vi "controleMF.vi"() -> ()   [LabVIEW 2019]
uses:
  <vilib>/Utility/error.llb/DialogType.ctl
  <vilib>/DAQmx/write.llb/DAQmx Write (Counter Frequency 1Chan 1Samp).vi
  <vilib>/DAQmx/create/channels.llb/DAQmx Create Channel (CO-Pulse Generation-Frequency).vi
  <vilib>/DAQmx/configure/timing.llb/DAQmx Timing (Implicit).vi
  <vilib>/DAQmx/miscellaneous.llb/DAQmx Fill In Error Info.vi
  <vilib>/addons/control/pid/pid.llb/PID (DBL).vi
  <vilib>/Utility/file.llb/Write Delimited Spreadsheet (string).vi
  <instrlib>/Agilent 34970/Agilent 34970.lvlib
  <resource>/objmgr/daqmx.rc
  <vilib>/addons/control/pid/NI_PID_pid.lvlib
panel:
  in  "SP:":dbl(slide)=25.0 min=0.0 max=0.0 scale=25.0..50.0
  out "MV":dbl(graph)
  in  "Ts":dbl=1.0
  out "PV":dbl
  out "Process variable and Setpoint":cluster{"initial PV":dbl, "SP:":dbl}(graph)
  in  "PID gains":T1={"proportional gain (Kc)"=39.6, "integral time (Ti, min)"=14.617, "derivative time (Td, min)"=0.0} {"derivative time (Td, min)" format="%.3f"; "integral time (Ti, min)" format="%.3f"; "proportional gain (Kc)" format="%.6f"}
  in  "Frequency":dbl=1.0 format="%.6f"
  out "Duty Cycle":sgl=0.1 min=0.1 max=99.9 format="%#_6f"
  in  "Forno_on":bool=TRUE
  out "Iteration":i32
  out "Chart PV, SP":cluster{dbl, dbl}(graph)
  in  "STOP":bool
  out "Temperature CH4 [degC]":dbl
  out "Temperature CH9 [degC]":dbl
  out "Time":dbl=300.0 format="%<%H:%M:%S>t"
  in  "Identifier":string="ensaioForno"
  # "Geral"
  # "Respostas do Sistema em Malha Fechada"
  # "Controles"
  # "Medidas"
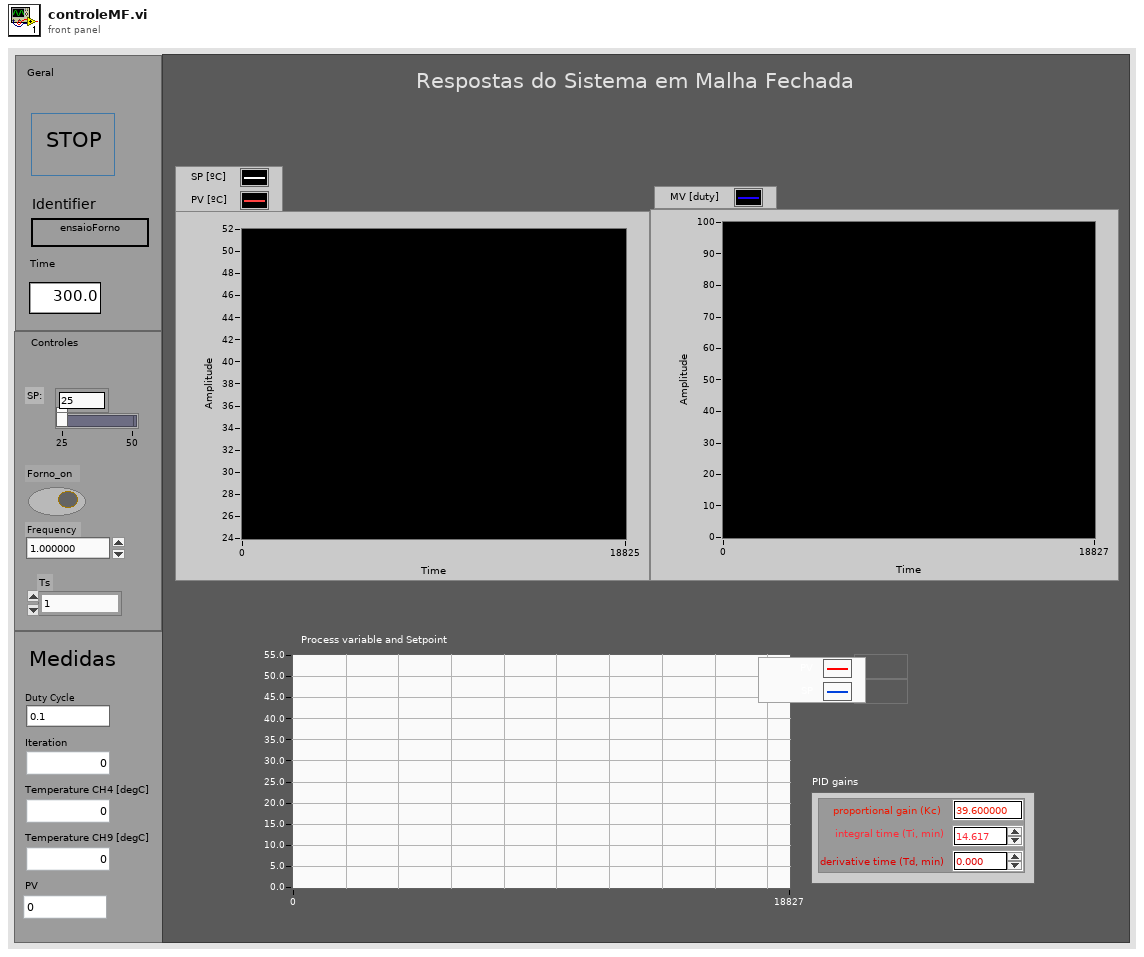
[diagram p1: front panel]
types:
  T1 = cluster{"proportional gain (Kc)":dbl, "integral time (Ti, min)":dbl, "derivative time (Td, min)":dbl}
  T2 = enum16{"Thermocouple", "Thermistor", "RTD", "4-Wire RTD", "Default (Last)"}
  T3 = typedef "DialogType.ctl" = u16
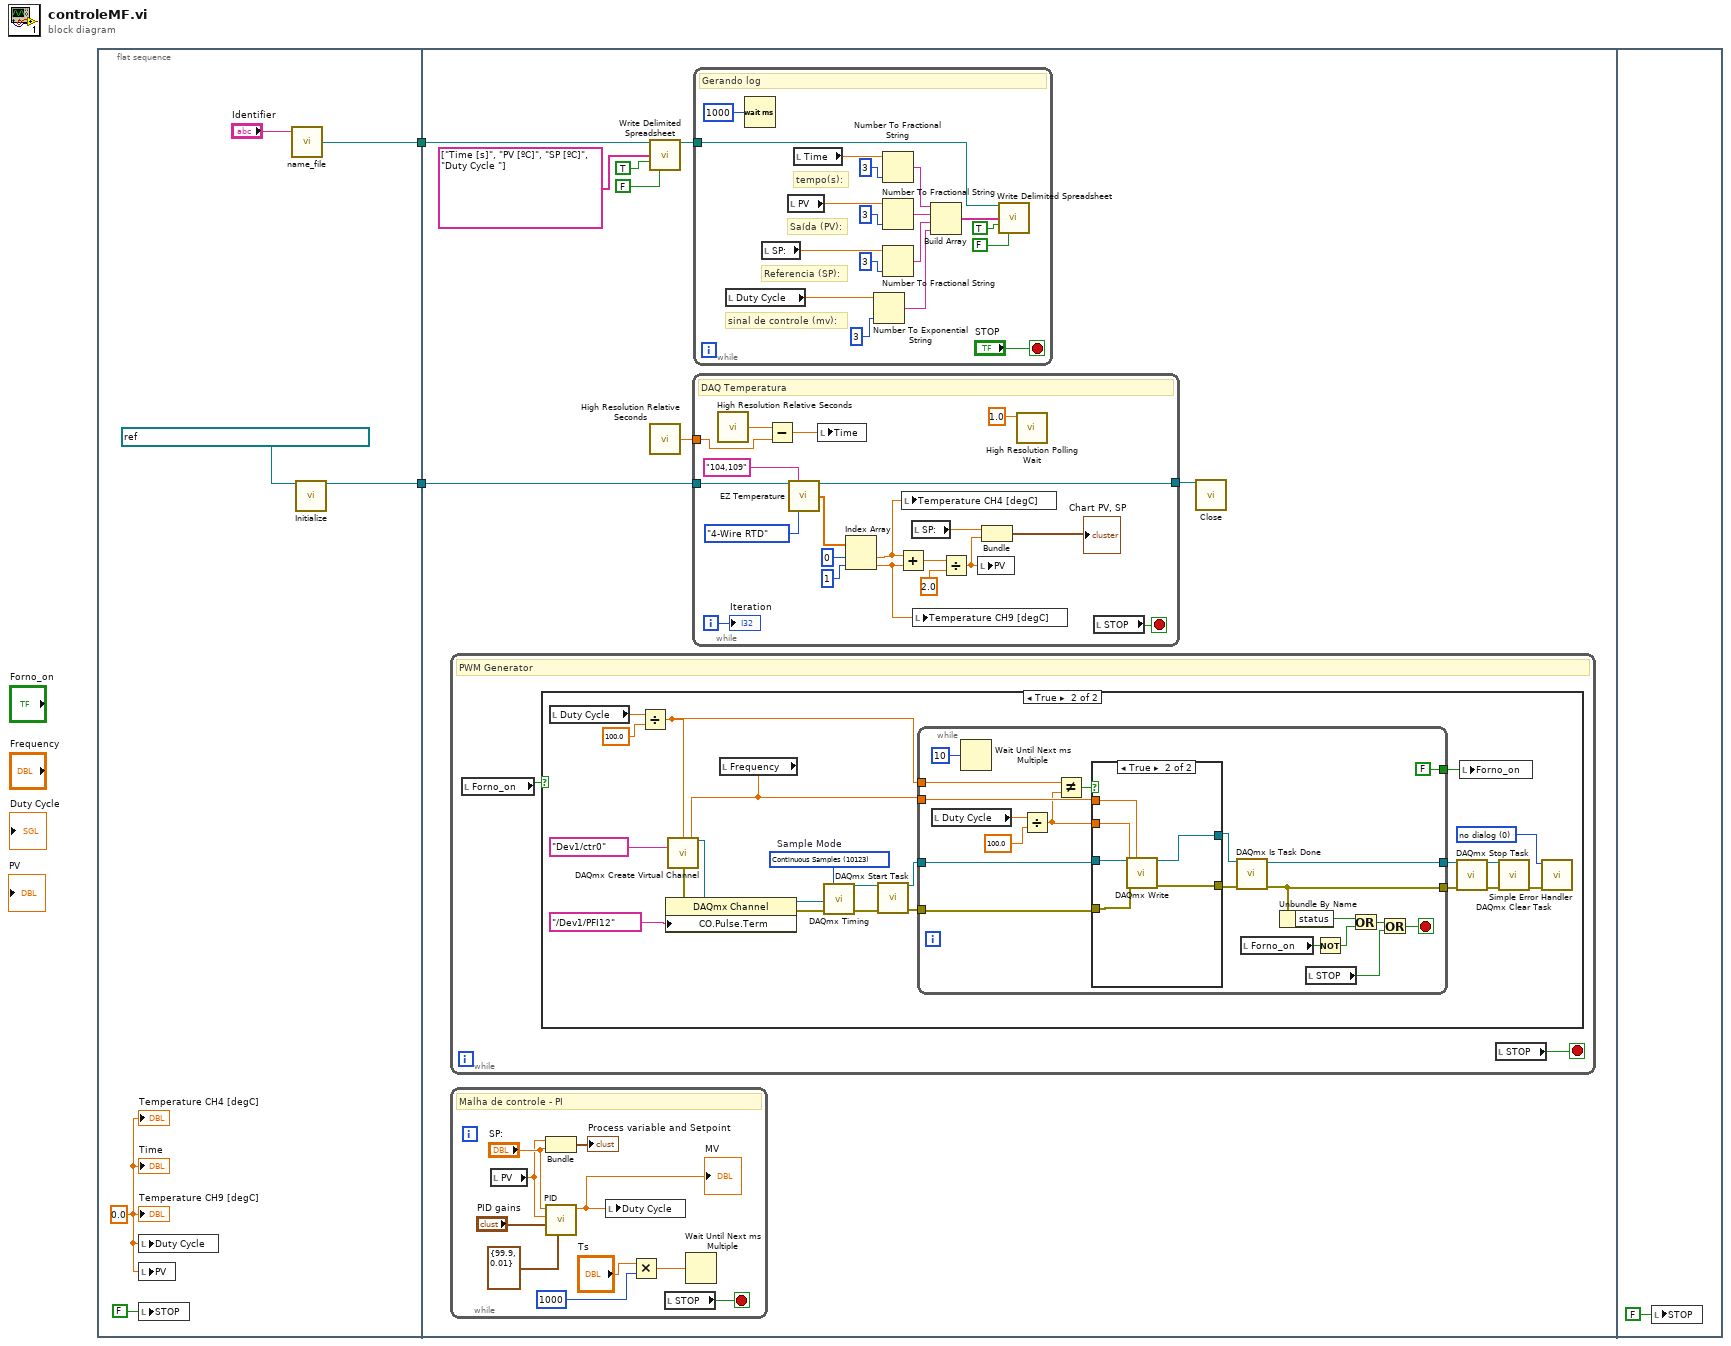
[diagram p0: block diagram]
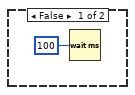
[diagram p2: hidden frame]
diagram:
  n1 = flat-sequence {
    tunnel: [w7] -> w2
    tunnel: [w6] -> w1
    tunnel: w2 -> [w14]
    tunnel: w1 -> [w9]
    frame #0 {
      w3 = 0.0 ("Temperature 1")
      n2 = local write "Duty Cycle"(w3) -> ()
      n3 = local write "PV"(w3) -> ()
      n4 = local write "STOP"(FALSE ("STOP")) -> ()
      n5 = call "name_file.vi"("Identifier"="Identifier") -> ("appended path"=w6:path)  [unwired: 2 in]
      n6 = call <instrlib>:"Initialize.vi"("VISA Resource Name"=refnum<visa-resource-name> "USB0::0x0957::0x2007::MY49006789::INSTR" ("VISA AGILENT")) -> ("VISA Resource Name Out"=w7:refnum<visa-resource-name>)  [unwired: 13 in, 1 out]
      "Temperature CH4 [degC]" <- w3
      "Temperature CH9 [degC]" <- w3
      "Time" <- w3
    }
    frame #1 {
      n7 = while {
        stop <- w27 stop-if-true
        # "PWM Generator"
        n8 = local read "Forno_on"() -> (w28:bool)
        n9 = case shown="True" w28 {
          frame False {
            n10 = Wait (ms)(milliseconds to wait=u32 100) -> ()  [unwired: 1 out]
          }
          frame True {
            w36 = T3 0 items=["no dialog", "OK message", "continue or stop message", "OK message + warnings", "continue/stop + warnings"] ("type of dialog (OK msg:1)")
            w47 = 10123 items=["Finite Samples"=10178, "Continuous Samples"=10123, "Hardware Timed Single Point"=12522]  # Sample Mode
            n11 = local read "Duty Cycle"() -> (w31:sgl)
            n12 = Divide(x=w31, y=100.0) -> (x/y=w30:dbl)
            n13 = local read "Frequency"() -> (w33:dbl)
            n14 = call-poly <vilib>:"DAQmx Create Virtual Channel.vi"("frequency"=w33, "duty cycle"=w30, "counter"=tag "Dev1/ctr0" ("Counter")) -> ("task out"=w50:refnum<k21>, "error out"=w49:errorcluster)  [unwired: 11 in]
            n15 = property class="DAQmx Channel"(reference=w50, error in=w49, "CO.Pulse.Term"=tag "/Dev1/PFI12" ("Output Terminal")) -> (reference out=w46:refnum<k21>, error out=w45:errorcluster)
            n16 = call-poly <vilib>:"DAQmx Timing.vi"("task/channels in"=w46, "sample mode"=w47, "error in"=w45) -> ("task out"=w44:refnum<k21>, "error out"=w43:errorcluster)  [unwired: 11 in]
            n17 = call <vilib>:"DAQmx Start Task.vi"("task/channels in"=w44, "error in"=w43) -> ("task out"=w42:refnum<k21>, "error out"=w41:errorcluster)  [unwired: 12 in]
            n18 = while {
              tunnel: w42 -> [w61]
              tunnel: w41 -> [w59]
              tunnel: [w70] -> w38
              tunnel: [w71] -> w39
              tunnel: [FALSE ("Liga aquecedor")] -> w35
              tunnel: w30 -> [w57]
              tunnel: w33 -> [w55]
              stop <- w64 stop-if-true
              n19 = local read "Duty Cycle"() -> (w54:sgl)
              n20 = Wait Until Next ms Multiple(millisecond multiple=u32 10) -> ()  [unwired: 1 out]
              n21 = Divide(x=w54, y=100.0) -> (x/y=w52:dbl)
              n22 = Not Equal?(x=w57, y=w52) -> (x != y?=w56:bool)
              n23 = case shown="True" w56 {
                tunnel: [w73 w76] -> w60
                tunnel: w61 -> [w73 w77]
                tunnel: [w72 w78] -> w58
                tunnel: w59 -> [w72 w79]
                tunnel: w52 -> [_ w75]
                tunnel: w55 -> [_ w74]
                frame False {
                }
                frame True {
                  n24 = call-poly <vilib>:"DAQmx Write.vi"("task/channels in"=w77, "frequency"=w74, "duty cycle"=w75, "error in"=w79) -> ("task out"=w76:refnum<k21>, "error out"=w78:errorcluster)  [unwired: 9 in, 1 out]
                }
              }
              n25 = call <vilib>:"DAQmx Is Task Done.vi"("task/channels in"=w60, "error in"=w58) -> ("task out"=w71:refnum<k21>, "error out"=w70:errorcluster)  [unwired: 11 in, 1 out]
              n26 = local read "Forno_on"() -> (w67:bool)
              n27 = Unbundle By Name(w70) -> ("status"=w69:bool)
              n28 = local read "STOP"() -> (w62:bool)
              n29 = Not(x=w67) -> (.not. x?=w65:bool)
              n30 = Or(x=w69, y=w65) -> (x .or. y?=w63:bool)
              n31 = Or(x=w63, y=w62) -> (x .or. y?=w64:bool)
            }
            n32 = call <vilib>:"DAQmx Stop Task.vi"("task/channels in"=w39, "error in"=w38) -> ("task out"=w34:refnum<k21>, "error out"=w40:errorcluster)  [unwired: 12 in]
            n33 = local write "Forno_on"(w35) -> ()
            n34 = call <vilib>:"DAQmx Clear Task.vi"("task in"=w34, "error in"=w40) -> ("error out"=w37:errorcluster)  [unwired: 13 in]
            n35 = call <vilib>:"Simple Error Handler.vi"("error code (no error:0)"=w36, "error in (no error)"=w37) -> ()  [unwired: 3 in, 5 out]
          }
        }
        n36 = local read "STOP"() -> (w27:bool)
      }
      n37 = while {
        stop <- w19 stop-if-true
        # "Malha de controle - PI"
        n38 = local read "PV"() -> (w23:dbl)
        n39 = Bundle("PV"=w23, "SP:"="SP:") -> (→"Process variable and Setpoint":cluster{"PV":dbl, "SP:":dbl})  [unwired: 1 in]
        n40 = call-poly <vilib>:"PID.vi"("output range"=cluster{"output high":dbl, "output low":dbl} {"output high"=99.9, "output low"=0.01}, "PID gains"="PID gains", "process variable"=w23, "setpoint"="SP:") -> ("output"=w18:dbl)  [unwired: 6 in, 1 out]
        "MV" <- w18
        n41 = local write "Duty Cycle"(w18) -> ()
        n42 = Multiply(x="Ts", y=u32 1000 ("unsigned 32bit integer")) -> (x*y=w17:dbl)
        n43 = local read "STOP"() -> (w19:bool)
        n44 = Wait Until Next ms Multiple(millisecond multiple=w17) -> ()  [unwired: 1 out]
      }
      n45 = call-poly <vilib>:"Write Delimited Spreadsheet.vi"("file path (dialog if empty)"=w9, "1D data"=string[] ["Time [s]", "PV [ºC]", "SP [ºC]", "Duty Cycle "] ("appended array"), "append to file? (new file:F)"=TRUE, "transpose? (no:F)"=FALSE) -> ("new file path (Not A Path if cancelled)"=w10:path)  [unwired: 10 in, 1 out]
      n46 = call <vilib>:"High Resolution Relative Seconds.vi"() -> ("relative seconds"=w16:dbl)
      n47 = while {
        tunnel: w14 -> [w113]
        tunnel: w16 -> [w114]
        tunnel: [w112] -> w15
        i -> [w116]
        stop <- w106 stop-if-true
        # "DAQ Temperatura"
        n48 = call <vilib>:"High Resolution Relative Seconds.vi"() -> ("relative seconds"=w115:dbl)
        n49 = Subtract(x=w115, y=w114) -> (x-y=w107:dbl)
        n50 = call <instrlib>:"EZ Temperature.vi"("VISA Resource Name"=w113, "Scan List (empty)"="104,109", "Transducer Type (4:Def-Last)"=T2."4-Wire RTD") -> ("VISA Resource Name Out"=w112:refnum<visa-resource-name>, "Output Array"=w105:dbl[])  [unwired: 10 in, 1 out]
        n51 = local write "Time"(w107) -> ()
        n52 = Index Array(array=w105, index #1=0 ("index"), index #2=1 ("index")) -> (element #1=w98:dbl, element #2=w99:dbl)
        n53 = Add(x=w98, y=w99) -> (x+y=w104:dbl)
        n54 = local write "Temperature CH4 [degC]"(w98) -> ()
        n55 = local read "SP:"() -> (w102:dbl)
        n56 = local write "Temperature CH9 [degC]"(w99) -> ()
        n57 = Divide(x=w104, y=2.0) -> (x/y=w101:dbl)
        n58 = local write "PV"(w101) -> ()
        n59 = Bundle("SP:"=w102, w101) -> (→"Chart PV, SP":cluster{"SP:":dbl, dbl})  [unwired: 1 in]
        n60 = call <vilib>:"High Resolution Polling Wait.vi"("seconds to wait"=1.0) -> ()  [unwired: 10 in, 1 out]
        n61 = local read "STOP"() -> (w106:bool)
        "Iteration" <- w116
      }
      n62 = while {
        tunnel: w10 -> [w95]
        stop <- "STOP" stop-if-true
        # "tempo(s):"
        # "Saída (PV):"
        # "Referencia (SP):"
        # "sinal de controle (mv):"
        # "Gerando log"
        n63 = local read "Duty Cycle"() -> (w91:sgl)
        n64 = Wait (ms)(milliseconds to wait=u32 1000) -> ()  [unwired: 1 out]
        n65 = local read "SP:"() -> (w84:dbl)
        n66 = local read "PV"() -> (w90:dbl)
        n67 = local read "Time"() -> (w88:dbl)
        n68 = Number To Exponential String(number=w91, precision (6)=i16 3) -> (E-format string=w93:string)  [unwired: 2 in]
        n69 = Number To Fractional String(number=w88, precision (6)=i16 3) -> (F-format string=w87:string)  [unwired: 2 in]
        n70 = Number To Fractional String(number=w90, precision (6)=i16 3) -> (F-format string=w86:string)  [unwired: 2 in]
        n71 = Number To Fractional String(number=w84, precision (6)=i16 3) -> (F-format string=w82:string)  [unwired: 2 in]
        n72 = Build Array(w87, w86, w82, w93) -> (w83:string[])
        n73 = call-poly <vilib>:"Write Delimited Spreadsheet.vi"("file path (dialog if empty)"=w95, "1D data"=w83, "append to file? (new file:F)"=TRUE, "transpose? (no:F)"=FALSE) -> ()  [unwired: 10 in, 2 out]
      }
      n74 = call <instrlib>:"Close.vi"("VISA Resource Name"=w15) -> ()  [unwired: 14 in, 1 out]
    }
    frame #2 {
      n75 = local write "STOP"(FALSE ("STOP")) -> ()
    }
  }
